vi "format_jv_file_data.vi"(9 "j-v metrics":string[](array[string]), 10 "j-v data":string[][](array[string])) -> (2 "file data":string[][](array[string]))   [LabVIEW 2016]
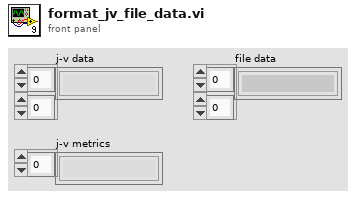
[diagram p1: front panel]
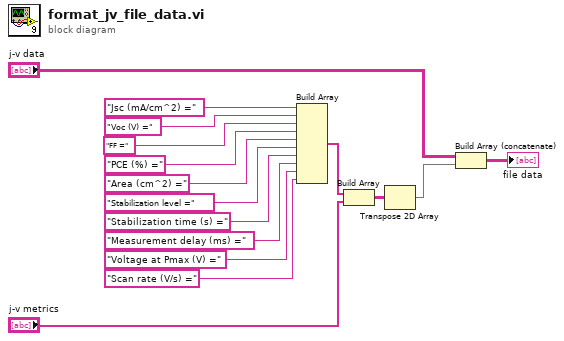
[diagram p0: block diagram]
diagram:
  n1 = Build Array("Jsc (mA/cm^2) =", "Voc (V) =", "FF =", "PCE (%) =", "Area (cm^2) =", "Stabilization level =", "Stabilization time (s) =", "Measurement delay (ms) =", "Voltage at Pmax (V) =", "Scan rate (V/s) =") -> (w5:string[])
  n2 = Build Array(w5, "j-v metrics") -> (w8:string[][])
  n3 = Transpose 2D Array(2D array=w8) -> (transposed array=w9:string[][])
  n4 = Build Array (concatenate)("j-v data", w9) -> (→"file data":string[][])
